vi "CustomStopService.vi"(8 "error in (no error)":errorcluster, 10 "Server Stop":refnum<user-event>, 11 "gRPC Server":refnum<class "Servicer.lvclass">) -> (0 "error out":errorcluster)   [LabVIEW 2019, in "MicronGRPCGeneratedServer.lvlib"]
uses:
  MicronGRPCGeneratedServer.lvlib
  <vilib>/gRPC/LabVIEW gRPC Servicer/Servicer/Servicer.lvclass
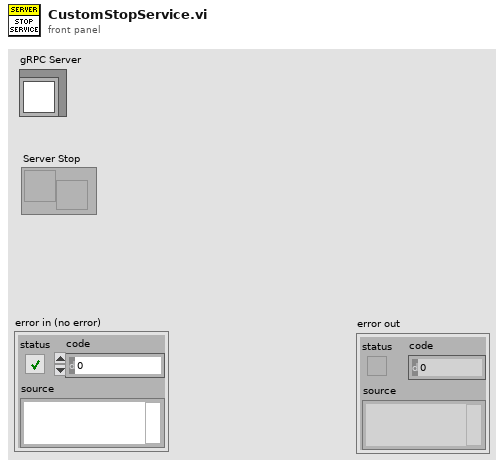
[diagram p1: front panel]
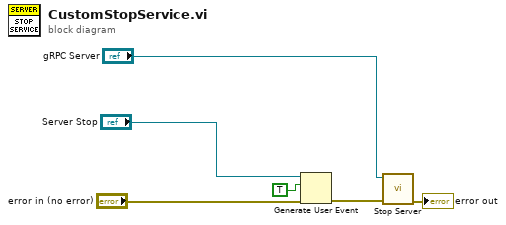
[diagram p0: block diagram]
diagram:
  n1 = Generate User Event(user event="Server Stop", event data cluster=TRUE ("event data"), error in="error in (no error)") -> (error out=w3:errorcluster)  [unwired: 1 in, 1 out]
  n2 = call <vilib>:"Stop Server.vi"("error in"=w3, "gRPC Server in"="gRPC Server") -> ("error out"=→"error out":errorcluster)  [unwired: 9 in]
